vi "Get Relay numbers 340-LEPL-103-A.vi"(8 "error in (no error)":errorcluster) -> (0 "error out":errorcluster, 2 "DUT2":T1, 3 "DUT1":T1)   [LabVIEW 2023]
uses:
  DUT_Relays_340-LEPL-103-A.ctl
  <vilib>/Utility/config.llb/Read Key (U32).vi
  <vilib>/Utility/config.llb/NI_LVConfig.lvlib
panel:
  out "error IO":errorcluster
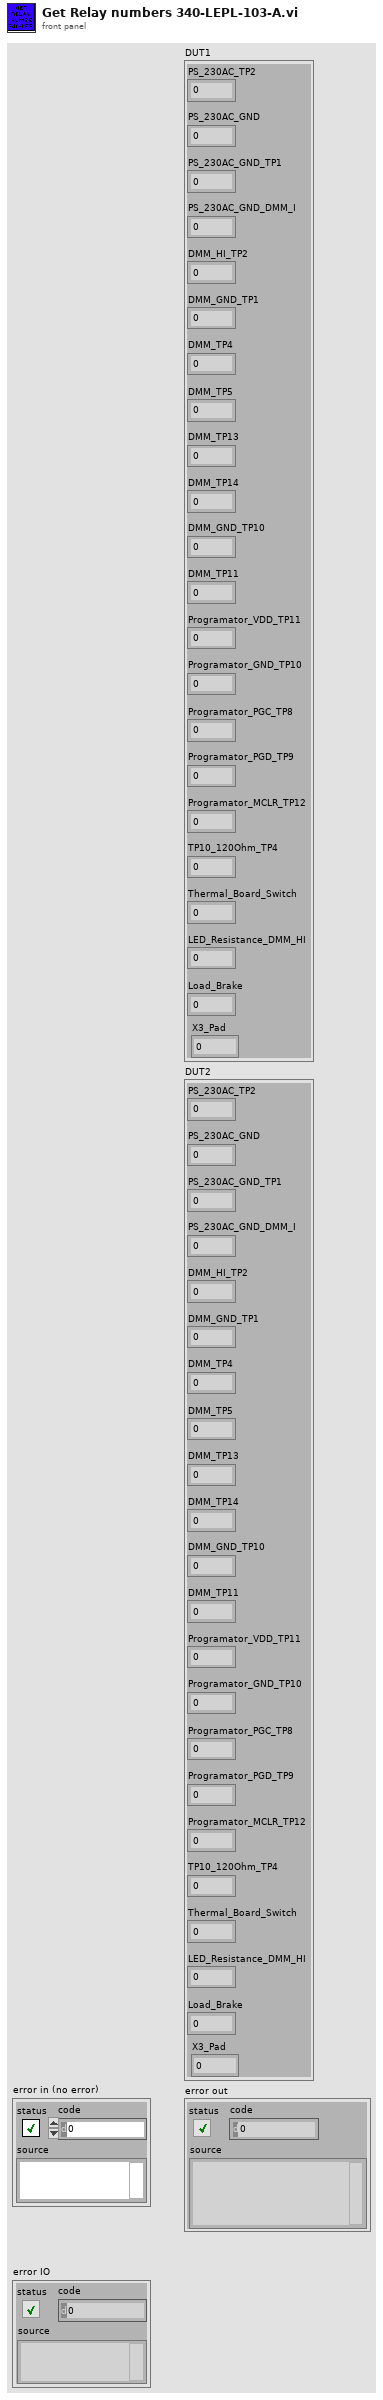
[diagram p1: front panel]
types:
  T1 = typedef "DUT_Relays_340-LEPL-103-A.ctl" = cluster{"PS_230AC_TP2":i32, "PS_230AC_GND":i32, "PS_230AC_GND_TP1":i32, "PS_230AC_GND_DMM_I":i32, "DMM_HI_TP2":i32, "DMM_GND_TP1":i32, "DMM_TP4":i32, "DMM_TP5":i32, "DMM_TP13":i32, "DMM_TP14":i32, "DMM_GND_TP10":i32, "DMM_TP11":i32, "Programator_VDD_TP11":i32, "Programator_GND_TP10":i32, "Programator_PGC_TP8":i32, "Programator_PGD_TP9":i32, "Programator_MCLR_TP12":i32, "TP10_120Ohm_TP4":i32, "Thermal_Board_Switch":i32, "LED_Resistance_DMM_HI":i32, "Load_Brake":i32, "X3_Pad":i32}
  T2 = typedef "NI_LVConfig.lvlib/Config Data RefNum.ctl" = refnum<k1>
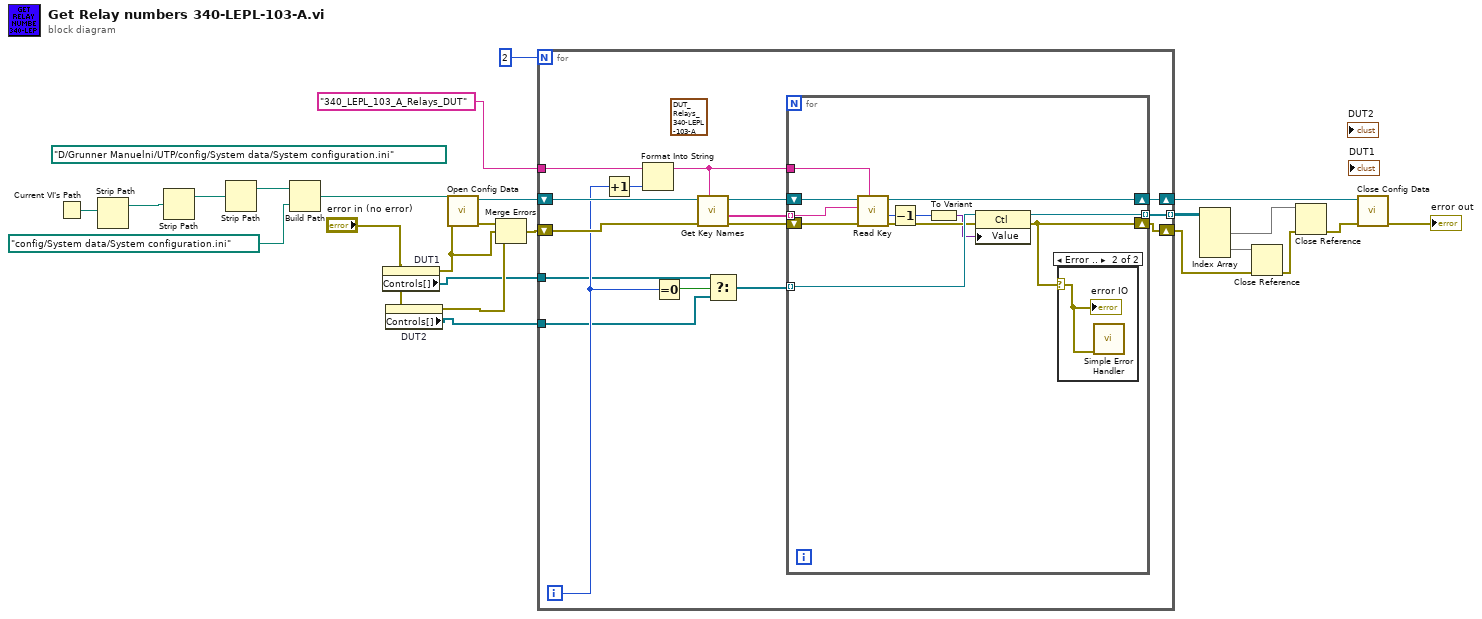
[diagram p0: block diagram]
diagram:
  (unwired) path "D:/Grunner Manuelni/UTP/config/System data/System configuration.ini" ("configuration file path")
  n1 = Current VI's Path() -> (path=w9:path)
  n2 = Strip Path(path=w9) -> (stripped path=w8:path)  [unwired: 1 out]
  n3 = Strip Path(path=w8) -> (stripped path=w12:path)  [unwired: 1 out]
  n4 = Strip Path(path=w12) -> (stripped path=w11:path)  [unwired: 1 out]
  n5 = Build Path(base path=w11, name or relative path=path "config/System data/System configuration.ini") -> (appended path=w7:path)
  n6 = property on="DUT1" class="Clust (strict)"(error in="error in (no error)") -> (error out=w1:errorcluster, "Controls[]"=w2:refnum<vi>[])  [unwired: 1 in, 1 out]
  n7 = property on="DUT2" class="Clust (strict)"(error in="error in (no error)") -> (error out=w5:errorcluster, "Controls[]"=w4:refnum<vi>[])  [unwired: 1 in, 1 out]
  n8 = call <vilib>:"Open Config Data.vi"("error in (no error)"=w1, "configuration file path"=w7) -> ("error out"=w18:errorcluster, "refnum"=w24:T2)  [unwired: 7 in, 1 out]
  n9 = Merge Errors(w18, w1, w5) -> (w19:errorcluster)
  n10 = for {
    N: 2 -> [_]
    shift-right: [w34] -> w23
    shift-left: w24 -> [w40]
    shift-right: [w35] -> w13
    shift-left: w19 -> [w37]
    tunnel: w2 -> [w30]
    tunnel: w4 -> [w27]
    tunnel: [w26] -> w17 mode=indexing
    tunnel: "340_LEPL_103_A_Relays_DUT" ("section") -> [w25]
    i -> [w31]
    (unwired) T1 {"PS_230AC_TP2"=0, "PS_230AC_GND"=0, "PS_230AC_GND_TP1"=0, "PS_230AC_GND_DMM_I"=0, "DMM_HI_TP2"=0, "DMM_GND_TP1"=0, "DMM_TP4"=0, "DMM_TP5"=0, "DMM_TP13"=0, "DMM_TP14"=0, "DMM_GND_TP10"=0, "DMM_TP11"=0, "Programator_VDD_TP11"=0, "Programator_GND_TP10"=0, "Programator_PGC_TP8"=0, "Programator_PGD_TP9"=0, "Programator_MCLR_TP12"=0, "TP10_120Ohm_TP4"=0, "Thermal_Board_Switch"=0, "LED_Resistance_DMM_HI"=0, "Load_Brake"=0, "X3_Pad"=0} ("DUT1 2")
    n11 = Increment(x=w31) -> (x+1=w33:i32)
    n12 = Format Into String(initial string=w25, w33) -> (resulting string=w32:string)  [unwired: 2 in, 1 out]
    n13 = Equal To 0?(x=w31) -> (x = 0?=w28:bool)
    n14 = call <vilib>:"Get Key Names.vi"("section"=w32, "error in (no error)"=w37, "refnum"=w40) -> ("error out"=w36:errorcluster, "key names"=w39:string[], "refnum out"=w38:T2)  [unwired: 5 in, 1 out]
    n15 = Select(t=w30, s=w28, f=w27) -> (s? t:f=w29:refnum<vi>[])
    n16 = for {
      tunnel: w39 -> [w50] mode=indexing
      shift-right: [w51] -> w34
      shift-left: w38 -> [w52]
      tunnel: w32 -> [w49]
      tunnel: w29 -> [w47] mode=indexing
      tunnel: [w43] -> w26 mode=indexing
      shift-right: [w42] -> w35
      shift-left: w36 -> [w48]
      n17 = call-poly <vilib>:"Read Key.vi"("section"=w49, "error in (no error)"=w48, "key"=w50, "refnum"=w52) -> ("error out"=w46:errorcluster, "value"=w45:u32, "refnum out"=w51:T2)  [unwired: 4 in, 1 out]
      n18 = Decrement(x=w45) -> (x-1=w41:u32)
      n19 = To Variant(anything=w41) -> (Variant=w44:variant)
      n20 = property class="Ctl"(reference=w47, error in=w46, "Value"=w44) -> (reference out=w43:refnum<vi>, error out=w42:errorcluster)
      n21 = case shown="Error .." w42 {
        selector: w42 -> [_ w53]
        frame No Error {
        }
        frame Error {
          n22 = call <vilib>:"Simple Error Handler.vi"("error in (no error)"=w53) -> ()  [unwired: 4 in, 5 out]
          "error IO" <- w53
        }
      }
    }
  }
  n23 = Index Array(array=w17) -> (element #1=w16:refnum<vi>[], element #2=w15:refnum<vi>[])  [unwired: 4 in]
  n24 = Close Reference(reference=w15, error in (no error)=w13) -> (error out=w14:errorcluster)
  n25 = Close Reference(reference=w16, error in (no error)=w14) -> (error out=w22:errorcluster)
  n26 = call <vilib>:"Close Config Data.vi"("error in (no error)"=w22, "refnum"=w23) -> ("error out"=→"error out":errorcluster)  [unwired: 8 in, 1 out]
